vi "Initialize2.vi"(8 "error in (no error)":errorcluster, 11 "Acquisition in":refnum<class "Acquisition.lvclass">) -> (0 "error out":errorcluster, 3 "Acquisition out":refnum<class "Acquisition.lvclass">)   [LabVIEW 2012]
uses:
  Comm/Stream/Stream.lvclass
  Acquisition.lvclass
  Channel/Channel.lvclass
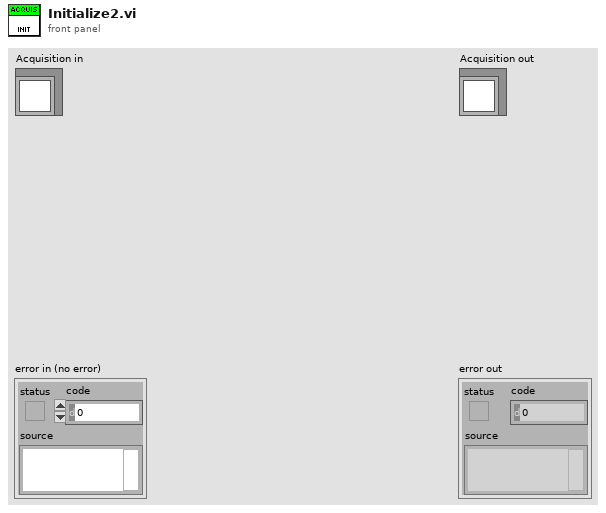
[diagram p1: front panel]
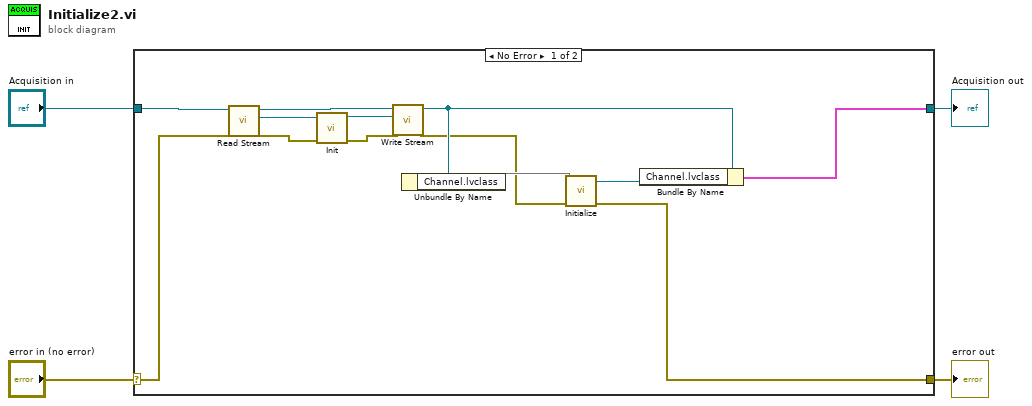
[diagram p0: block diagram]
diagram:
  n1 = case shown="No Error" "error in (no error)" {
    selector: "error in (no error)" -> [w9 w19]
    tunnel: [w14 w19] -> w3
    tunnel: [w17 w18] -> w2
    tunnel: "Acquisition in" -> [w5 w18]
    frame No Error {
      n2 = call-dynamic "Read Stream.vi"("error in (no error)"=w9, "Server in"=w5) -> ("error out"=w8:errorcluster, "Stream.lvclass"=w13:refnum<class "Stream.lvclass">, "Server out"=w12:refnum<class "Acquisition.lvclass">)  [unwired: 7 in]
      n3 = call-dynamic "Init.vi"("error in (no error)"=w8, "Stream in"=w13) -> ("error out"=w7:errorcluster, "Stream out"=w10:refnum<class "Stream.lvclass">)  [unwired: 8 in]
      n4 = call-dynamic "Write Stream.vi"("error in (no error)"=w7, "Stream.lvclass"=w10, "Server in"=w12) -> ("error out"=w6:errorcluster, "Server out"=w11:refnum<class "Acquisition.lvclass">)  [unwired: 7 in]
      n5 = Unbundle By Name(w11) -> ("Channel.lvclass"=w16)
      n6 = call-dynamic "Initialize.vi"("error in (no error)"=w6, "Channel in"=w16) -> ("error out"=w14:errorcluster, "Channel out"=w15:refnum<class "Channel.lvclass">)  [unwired: 8 in]
      n7 = Bundle By Name(cluster=w11, "Channel.lvclass"=w15) -> (w17:cluster{})
    }
    frame Error {
    }
  }
  "error out" <- w3
  "Acquisition out" <- w2
